vi "Temp_Sensor_Filter_subVI.vi"(10 "Temp Data In":cluster{dbl, dbl, dbl}, 11 "Apply Moving Average?":bool) -> (1 "T Write":T1, 2 "T Plot":T1, 3 "dT/dt Write":cluster{"dx/dt":dbl, "dx/dt":dbl, "dx/dt":dbl}, 4 "dT/dt Plot":cluster{"dx/dt":dbl, "dx/dt":dbl, "dx/dt":dbl})   [LabVIEW 2015]
uses:
  <vilib>/ptbypt/NI_PtbyPt.lvlib
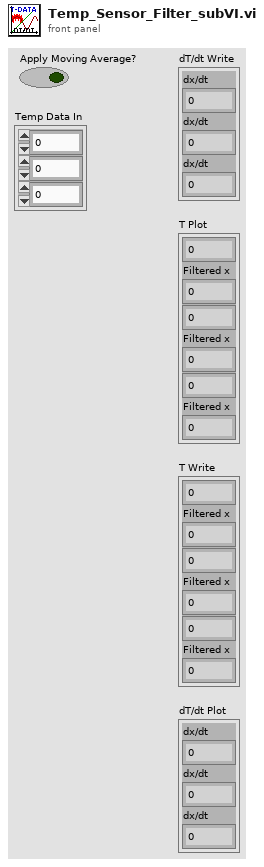
[diagram p1: front panel]
types:
  T1 = cluster{dbl, "Filtered x":dbl, dbl, "Filtered x":dbl, dbl, "Filtered x":dbl}
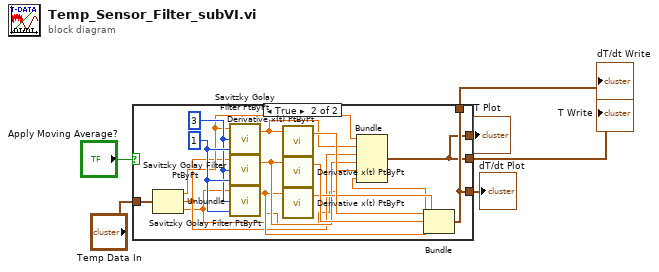
[diagram p0: block diagram]
diagram:
  n1 = case shown="True" "Apply Moving Average?" {
    tunnel: "Temp Data In" -> [_ w20]
    tunnel: [_ w7] -> w3
    tunnel: [_ w8] -> w4
    tunnel: [_ w8] -> w5
    tunnel: [_ w7] -> w6
    frame False {
    }
    frame True {
      w18 = 3 ("side points")
      w19 = 1 ("polynomial order")
      n2 = Unbundle(w20) -> (w14:dbl, w10:dbl, w9:dbl)
      n3 = call <vilib>:"Savitzky Golay Filter PtByPt.vi"("order polynomial"=w19, "side points"=w18, "x"=w14) -> ("Filtered x"=w13:dbl)  [unwired: 1 in, 1 out]
      n4 = call <vilib>:"Savitzky Golay Filter PtByPt.vi"("order polynomial"=w19, "side points"=w18, "x"=w10) -> ("Filtered x"=w12:dbl)  [unwired: 1 in, 1 out]
      n5 = call <vilib>:"Savitzky Golay Filter PtByPt.vi"("order polynomial"=w19, "side points"=w18, "x"=w9) -> ("Filtered x"=w11:dbl)  [unwired: 1 in, 1 out]
      n6 = call <vilib>:"Derivative x(t) PtByPt.vi"("x"=w13) -> ("dx/dt"=w17:dbl)  [unwired: 3 in, 1 out]
      n7 = call <vilib>:"Derivative x(t) PtByPt.vi"("x"=w12) -> ("dx/dt"=w16:dbl)  [unwired: 3 in, 1 out]
      n8 = call <vilib>:"Derivative x(t) PtByPt.vi"("x"=w11) -> ("dx/dt"=w15:dbl)  [unwired: 3 in, 1 out]
      n9 = Bundle(w14, "Filtered x"=w13, w10, "Filtered x"=w12, w9, "Filtered x"=w11) -> (w7:T1)  [unwired: 1 in]
      n10 = Bundle("dx/dt"=w17, "dx/dt"=w16, "dx/dt"=w15) -> (w8:cluster{"dx/dt":dbl, "dx/dt":dbl, "dx/dt":dbl})  [unwired: 1 in]
    }
  }
  "T Plot" <- w6
  "dT/dt Plot" <- w5
  "dT/dt Write" <- w4
  "T Write" <- w3
